vi "VIPM to NIPM - Wrapper Converter.vi"() -> ()   [LabVIEW 2016]
uses:
  support/dependencies.ctl
  vipm-to-nipm-package-converter.lvlib
  <vilib>/JKI/VIPM API/VIPM API_vipm_api.lvlib
panel:
  out "Array 2":errorcluster[](array[cluster])
  out "Generated NIPM package (.nipkg)":path[](array[path])
  out "Array":T1[](array[typedef])
  out "error out":errorcluster
  in  "Destination folder":path
  in  "error in (no error)":errorcluster
  in  "Source VIPM package (.vip)":path
  # "e.g. \"14.0\", \"14.0 (64-bit)\", \"18.0\", \"18.0 (64-bit)\""
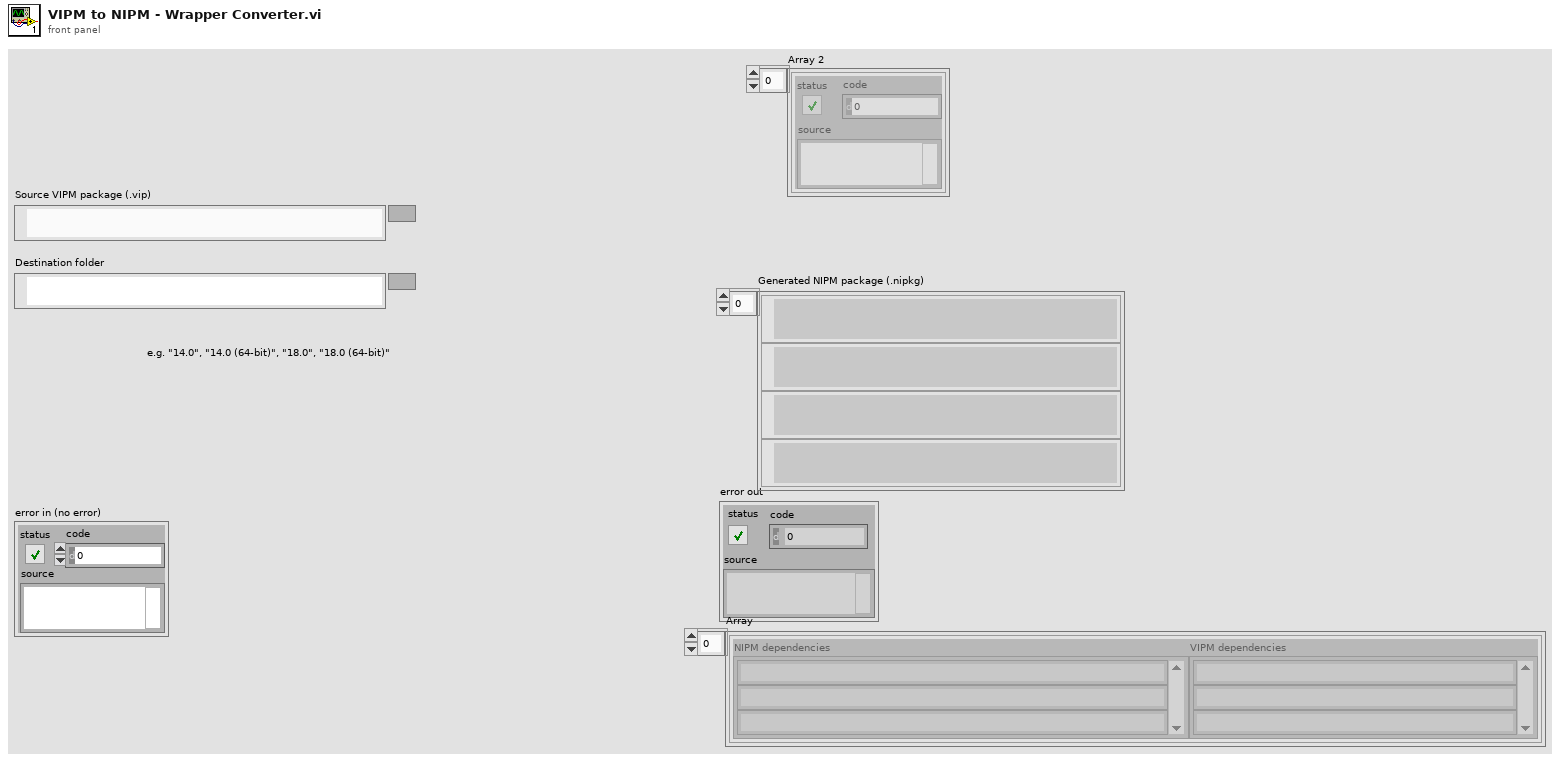
[diagram p1: front panel]
types:
  T1 = typedef "vipm-to-nipm-package-converter.lvlib/dependencies.ctl" = cluster{"NIPM dependencies":string[], "VIPM dependencies":string[]}
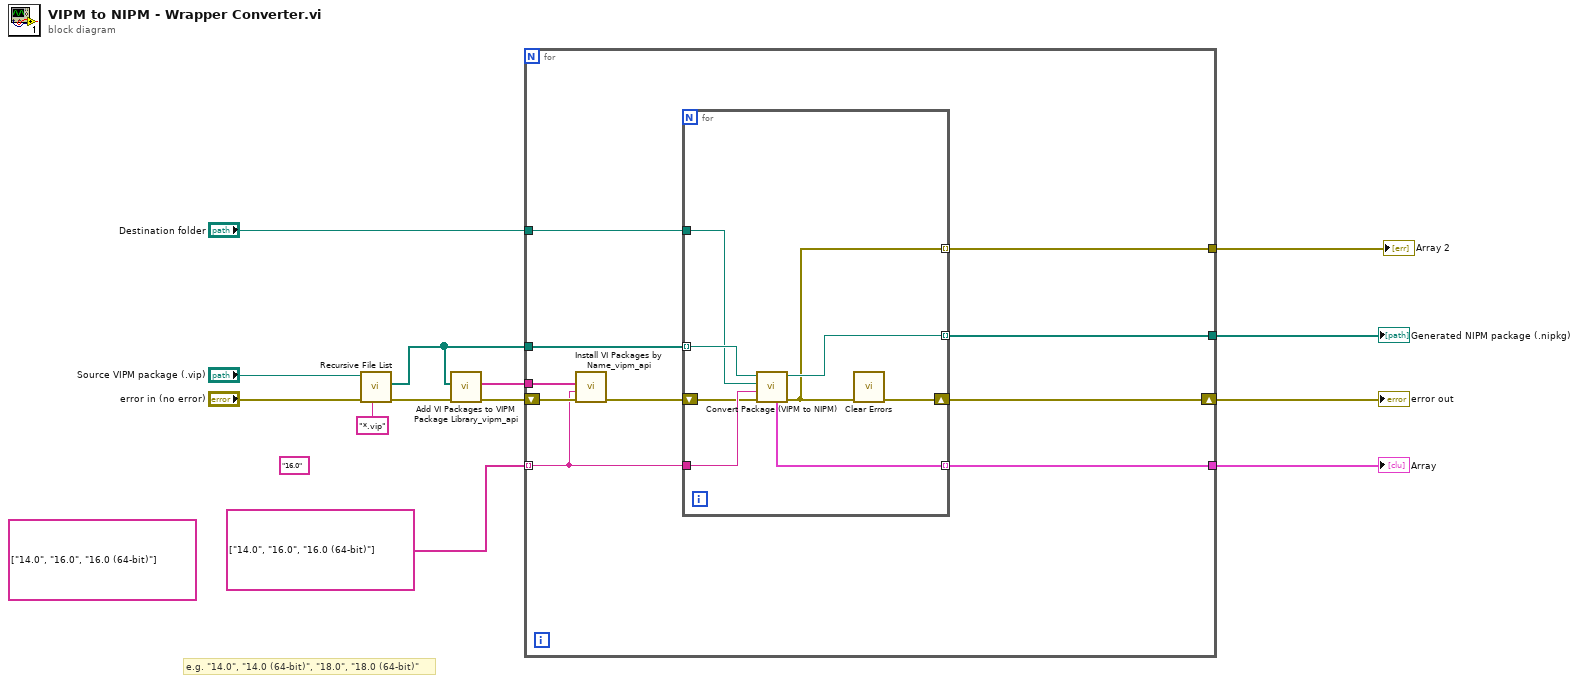
[diagram p0: block diagram]
diagram:
  (unwired) string[] ["14.0", "16.0", "16.0 (64-bit)"]
  (unwired) "16.0" ("LabVIEW version")
  # "e.g. \"14.0\", \"14.0 (64-bit)\", \"18.0\", \"18.0 (64-bit)\""
  n1 = call <vilib>:"Recursive File List.vi"("pattern"="*.vip", "error in (no error)"="error in (no error)", "Folder Path"="Source VIPM package (.vip)") -> ("error out"=w5:errorcluster, "All Files in Dir"=w4:path[])  [unwired: 4 in, 3 out]
  n2 = call <vilib>:"Add VI Packages to VIPM Package Library_vipm_api.vi"("error in (no error)"=w5, "Packages to add to VIPM Library (vipc,vip,ogp)"=w4) -> ("error out"=w3:errorcluster, "Package Names Added"=w2:string[])  [unwired: 8 in]
  n3 = for {
    tunnel: "Destination folder" -> [w22]
    tunnel: [w21] -> w8
    tunnel: [w20] -> w7
    tunnel: [w19] -> w6
    tunnel: w4 -> [w18]
    tunnel: w2 -> [w15]
    tunnel: string[] ["14.0", "16.0", "16.0 (64-bit)"] -> [w14] mode=indexing
    shift-right: [w23] -> w13
    shift-left: w3 -> [w17]
    n4 = call <vilib>:"Install VI Packages by Name_vipm_api.vi"("error in (no error)"=w17, "LabVIEW Version"=w14, "Package Names to Install []"=w15) -> ("error out"=w16:errorcluster)  [unwired: 8 in]
    n5 = for {
      shift-right: [w26] -> w23
      shift-left: w16 -> [w24]
      tunnel: w18 -> [w31] mode=indexing
      tunnel: w22 -> [w30]
      tunnel: [w29] -> w21 mode=indexing
      tunnel: [w28] -> w20 mode=indexing
      tunnel: [w27] -> w19 mode=indexing
      tunnel: w14 -> [w25]
      n6 = call "Convert Package (VIPM to NIPM).vi"("error in (no error)"=w24, "LabVIEW version"=w25, "Destination folder"=w30, "Source VIPM package (.vip)"=w31) -> ("error out"=w27:errorcluster, "Generated NIPM package (.nipkg)"=w28:path, "Dependencies"=w29:T1)  [unwired: 5 in]
      n7 = call <vilib>:"Clear Errors.vi"("error in (no error)"=w27) -> ("error out"=w26:errorcluster)  [unwired: 5 in, 1 out]
    }
  }
  "error out" <- w13
  "Array" <- w8
  "Generated NIPM package (.nipkg)" <- w7
  "Array 2" <- w6
